vi "Create Memento.vi"(8 "error in (no error)":errorcluster, 11 "IMementoNumeric in":refnum<class "IMementoNumeric.lvclass">) -> (0 "error out":errorcluster, 2 "Numeric Memento":refnum<class>, 3 "IMementoNumeric out":refnum<class "IMementoNumeric.lvclass">)   [LabVIEW 2009, in "IMementoNumeric.lvclass"]
uses:
  IMementoNumeric.lvclass
  Numeric Test Object.lvclass
  MementoNumeric/MementoNumeric.lvclass
  Source/IUnknown Class/IUnknown.lvclass
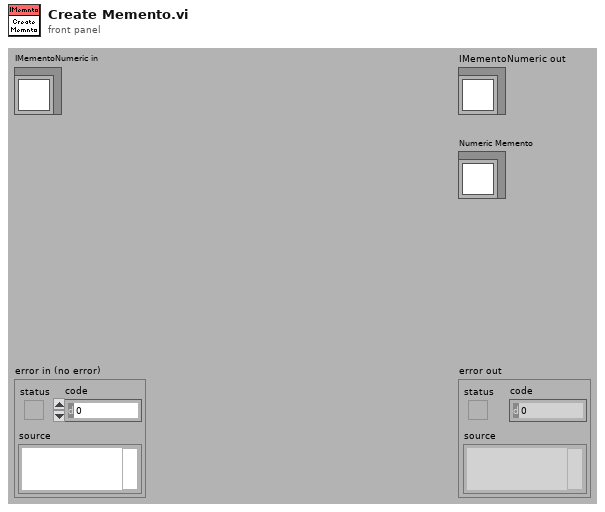
[diagram p1: front panel]
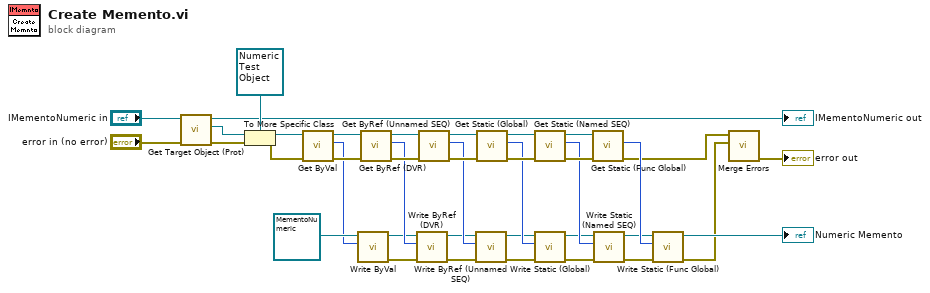
[diagram p0: block diagram]
diagram:
  n1 = call "Get Target Object (Prot).vi"("error in (no error)"="error in (no error)", "IUnknown in"="IMementoNumeric in") -> ("error out"=w35:errorcluster, "Target Object"=w37:refnum<class "Interfaceable.lvclass">, "IUnknown out"=→"IMementoNumeric out":refnum<class "IMementoNumeric.lvclass">)  [unwired: 7 in]
  n2 = To More Specific Class(target class=refnum<class "Numeric Test Object.lvclass"> refnum ("Numeric"), reference=w37, error in=w35) -> (specific class reference=w22:refnum<class "Numeric Test Object.lvclass">, error out=w21:errorcluster)
  n3 = call-dynamic "Get ByVal.vi"("error in (no error)"=w21, "Numeric in"=w22) -> ("error out"=w30:errorcluster, "Int"=w20:i32, "Numeric out"=w34:refnum<class "Numeric Test Object.lvclass">)  [unwired: 7 in]
  n4 = call "Write ByVal.vi"("ByVal"=w20, "MementoNumeric in"=refnum<class "MementoNumeric.lvclass"> refnum ("MementoNumeric")) -> ("error out"=w5:errorcluster, "MementoNumeric out"=w14:refnum<class "MementoNumeric.lvclass">)  [unwired: 8 in]
  n5 = call-dynamic "Get ByRef (DVR).vi"("error in (no error)"=w30, "Numeric in"=w34) -> ("error out"=w29:errorcluster, "Int"=w19:i32, "Numeric out"=w33:refnum<class "Numeric Test Object.lvclass">)  [unwired: 7 in]
  n6 = call "Write ByRef (DVR).vi"("error in (no error)"=w5, "ByRef (DVR)"=w19, "MementoNumeric in"=w14) -> ("error out"=w4:errorcluster, "MementoNumeric out"=w13:refnum<class "MementoNumeric.lvclass">)  [unwired: 7 in]
  n7 = call-dynamic "Get ByRef (Unnamed SEQ).vi"("error in (no error)"=w29, "Numeric in"=w33) -> ("error out"=w28:errorcluster, "Int"=w18:i32, "Numeric out"=w32:refnum<class "Numeric Test Object.lvclass">)  [unwired: 7 in]
  n8 = call "Write ByRef (Unnamed SEQ).vi"("error in (no error)"=w4, "ByRef (Unnamed SEQ)"=w18, "MementoNumeric in"=w13) -> ("error out"=w3:errorcluster, "MementoNumeric out"=w12:refnum<class "MementoNumeric.lvclass">)  [unwired: 7 in]
  n9 = call-dynamic "Get Static (Global).vi"("error in (no error)"=w28, "Numeric in"=w32) -> ("error out"=w27:errorcluster, "Int"=w17:i32, "Numeric out"=w31:refnum<class "Numeric Test Object.lvclass">)  [unwired: 7 in]
  n10 = call-dynamic "Get Static (Named SEQ).vi"("error in (no error)"=w27, "Numeric in"=w31) -> ("error out"=w23:errorcluster, "Int"=w16:i32, "Numeric out"=w24:refnum<class "Numeric Test Object.lvclass">)  [unwired: 7 in]
  n11 = call "Write Static (Global).vi"("error in (no error)"=w3, "Static (Global)"=w17, "MementoNumeric in"=w12) -> ("error out"=w2:errorcluster, "MementoNumeric out"=w11:refnum<class "MementoNumeric.lvclass">)  [unwired: 7 in]
  n12 = call-dynamic "Get Static (Func Global).vi"("error in (no error)"=w23, "Numeric in"=w24) -> ("error out"=w8:errorcluster, "Int"=w15:i32)  [unwired: 7 in, 1 out]
  n13 = call "Write Static (Named SEQ).vi"("error in (no error)"=w2, "Static (Named SEQ)"=w16, "MementoNumeric in"=w11) -> ("error out"=w1:errorcluster, "MementoNumeric out"=w10:refnum<class "MementoNumeric.lvclass">)  [unwired: 7 in]
  n14 = call "Write Static (Func Global).vi"("error in (no error)"=w1, "Static (Func Global)"=w15, "MementoNumeric in"=w10) -> ("error out"=w7:errorcluster, "MementoNumeric out"=→"Numeric Memento":refnum<class "MementoNumeric.lvclass">)  [unwired: 7 in]
  n15 = call <vilib>:"Merge Errors.vi"("error in 2 (no error)"=w7, "error in 1 (no error)"=w8) -> ("error out"=→"error out":errorcluster)  [unwired: 5 in]
